vi "1204_FirstLabview.vi"() -> ()   [LabVIEW 2018]
panel:
  out "불리언 3":bool
  in  "불리언 2":bool
  in  "불리언":bool
  in  "노브":dbl(knob) scale=0.0..10.0
  out "곱셈 결과":dbl
  out "더하기":dbl
  in  "숫자형 2":dbl
  in  "숫자형":dbl
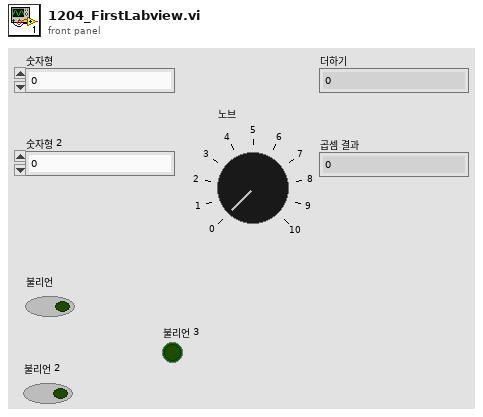
[diagram p1: front panel]
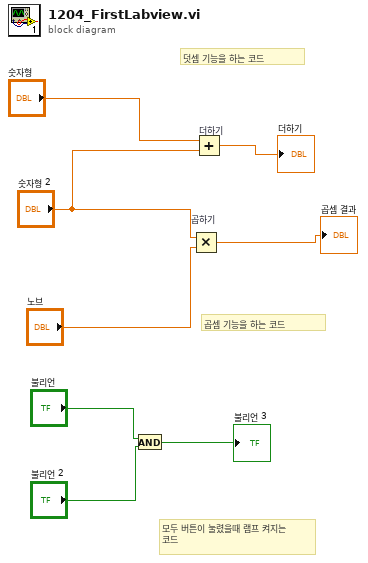
[diagram p0: block diagram]
diagram:
  # "모두 버튼이 눌렸을때 램프 켜지는 코드"
  # "곱셈 기능을 하는 코드"
  # "덧셈 기능을 하는 코드"
  n1 = And(x="불리언", y="불리언 2") -> (x .and. y?=→"불리언 3":bool)
  n2 = Multiply "곱하기"(x="숫자형 2", y="노브") -> (x*y=→"곱셈 결과":dbl)
  n3 = Add "더하기"(x="숫자형", y="숫자형 2") -> (x+y=→"더하기":dbl)
